vi "AnalyseAllFITSPlanes.vi"(3 "error in":errorcluster, 5 "file path":path=path "D:/freigabe/raw_I000_X0_C3_ministack.fits") -> (0 "error out":errorcluster, 2 "Mean,std,slope,min,max":dbl[](array[numeric]))   [LabVIEW 2011]
uses:
  <vilib>/Analysis/NI_AALBase.lvlib
  <vilib>/Analysis/NI_AALPro.lvlib
panel:
  out "Array":dbl[][](array[numeric])
  out "Mean Chart":dbl(graph)=34.04643333333333
  out "Intensity Graph":sgl[][](graph)
  out "FITS":T1={"BITPIX"=16, "NAXIS"=3, "NAXIS1"=300, "NAXIS2"=300, "NAXIS3"=168, "BZERO"=32768.0, "BSCALE"=1.0}
  # "this is IJ-Orientation"
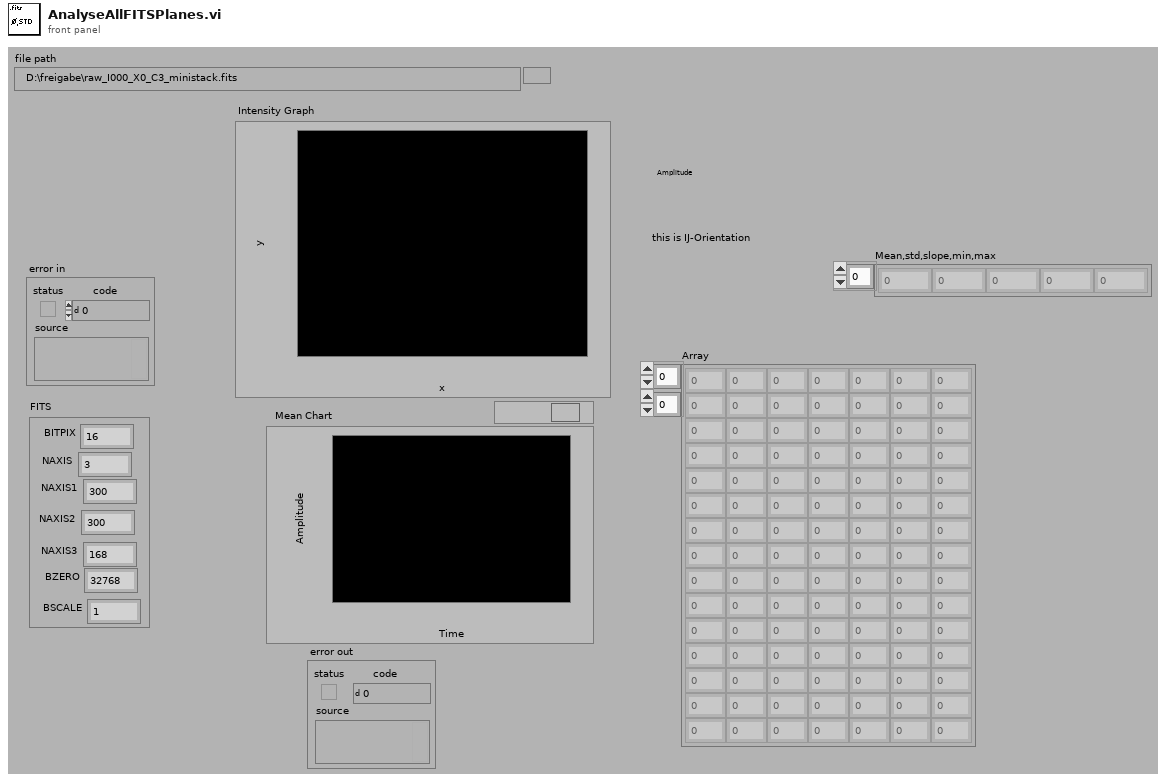
[diagram p1: front panel]
types:
  T1 = cluster{"BITPIX":i16, "NAXIS":i16, "NAXIS1":u16, "NAXIS2":u16, "NAXIS3":u16, "BZERO":dbl, "BSCALE":dbl}
  T2 = cluster{"fits refnum":refnum<file>, "Byte-Reihenfolge (0:Big-Endian, 2:LSB)":enum16{"big-endian, network order", "native, host order", "little-endian"}}
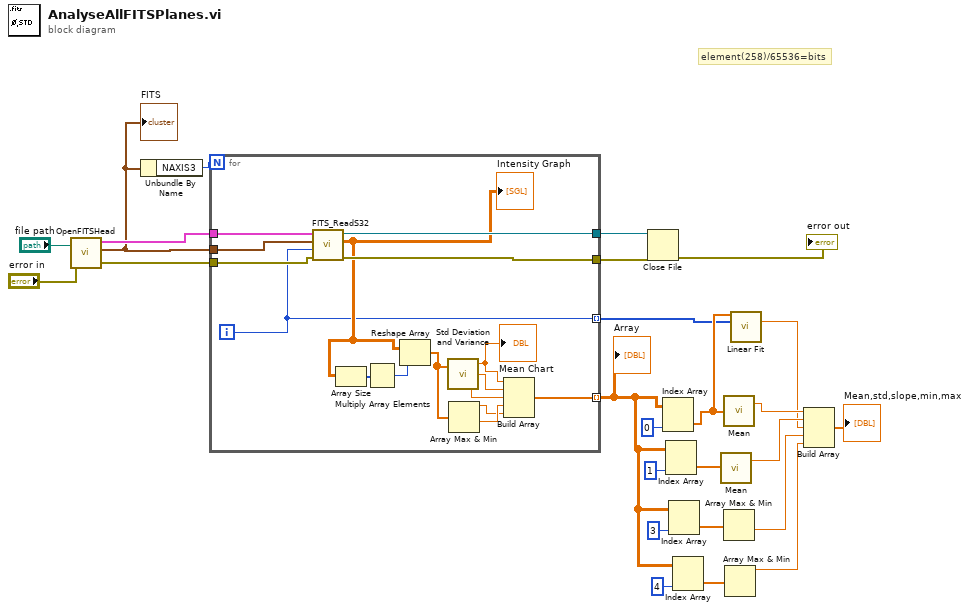
[diagram p0: block diagram]
diagram:
  # "element(258)/65536=bits"
  n1 = call "OpenFITSHead.vi"("file path"="file path", "error in"="error in") -> ("FITS file"=w22:T2, "FITS"=w20:T1, "error out"=w21:errorcluster)  [unwired: 1 in]
  "FITS" <- w20
  n2 = Unbundle By Name(w20) -> ("NAXIS3"=w19:u16)
  n3 = for {
    N: w19 -> [_]
    tunnel: w22 -> [w41]
    tunnel: w20 -> [w40]
    tunnel: w21 -> [w39]
    tunnel: [w38] -> w17
    tunnel: [w37] -> w18
    tunnel: [w29] -> w11 mode=indexing
    tunnel: [w26] -> w1 mode=indexing
    i -> [w26]
    n4 = call "FITS_ReadS32.vi"("error in (no error)"=w39, "Plane# (0..n-1)"=w26, "FITS"=w40, "FITS file"=w41) -> ("error out"=w38:errorcluster, "Array"=w36:sgl[][], "Byte Stream File out"=w37:refnum<file>)  [unwired: 5 in]
    "Intensity Graph" <- w36
    n5 = Array Size(array=w36) -> (size(s)=w35:i32[])
    n6 = Multiply Array Elements(1:w35) -> (0:w34:i32)
    n7 = Reshape Array(w36, w34) -> (w33:sgl[])
    n8 = call <vilib>:"Std Deviation and Variance.vi"("X"=w33) -> ("mean"=w32:dbl, "standard deviation"=w31:dbl, "variance"=w30:dbl)  [unwired: 1 in]
    "Mean Chart" <- w32
    n9 = Array Max & Min(array=w33) -> (max value=w27:sgl, min value=w28:sgl)  [unwired: 2 out]
    n10 = Build Array(w32, w31, w30, w28, w27) -> (w29:dbl[])
  }
  "Array" <- w11
  n11 = Close File(refnum=w18, error in=w17) -> (error out=→"error out":errorcluster)  [unwired: 1 out]
  n12 = Index Array(array=w11, index (col)=0 ("disabled index (col)")) -> (element=w3:dbl[])  [unwired: 1 in]
  n13 = Index Array(array=w11, index (col)=1 ("disabled index (col)")) -> (element=w14:dbl[])  [unwired: 1 in]
  n14 = Index Array(array=w11, index (col)=3 ("disabled index (col)")) -> (element=w12:dbl[])  [unwired: 1 in]
  n15 = Index Array(array=w11, index (col)=4 ("disabled index (col)")) -> (element=w9:dbl[])  [unwired: 1 in]
  n16 = call <vilib>:"Mean.vi"("X"=w14) -> ("mean"=w7:dbl)  [unwired: 1 out]
  n17 = call <vilib>:"Mean.vi"("X"=w3) -> ("mean"=w8:dbl)  [unwired: 1 out]
  n18 = Array Max & Min(array=w12) -> (min value=w6:dbl)  [unwired: 3 out]
  n19 = Array Max & Min(array=w9) -> (max value=w5:dbl)  [unwired: 3 out]
  n20 = call <vilib>:"Linear Fit.vi"("Y"=w3, "X"=w1) -> ("slope"=w2:dbl)  [unwired: 9 in, 4 out]
  n21 = Build Array(w8, w7, w2, w6, w5) -> (→"Mean,std,slope,min,max":dbl[])
